vi "GT Get Sts Ext Mdl.vi"(7 "pStatus":u16, 8 "error in (no error)":errorcluster caption="错误输入（无错误）", 9 "chn":i16, 10 "mdl":i16, 11 "cardNum":i16) -> (0 "error out":errorcluster caption="错误输出", 3 "function return":i16, 5 "pStatus out":u16)   [LabVIEW 2014, in "gts.lvlib"]
doc: "GT_API GT_GetStsExtMdl(short cardNum,short mdl,short chn,unsigned short *pStatus);"
uses:
  gts.lvlib
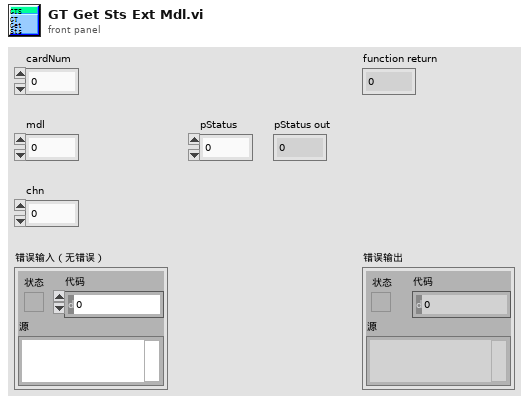
[diagram p1: front panel]
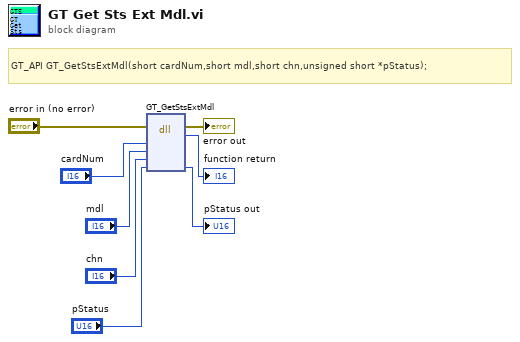
[diagram p0: block diagram]
diagram:
  # "GT_API GT_GetStsExtMdl(short cardNum,short mdl,short chn,unsigned short *pStatus);"
  n1 = dll-call lib="PTH2habs D固高科技资料GTS控制卡GTS卡18年上半年资料dllVC32bit\nmulti_cardgts.*" fn="GT_GetStsExtMdl"(error in="error in (no error)", "cardNum"="cardNum", "mdl"="mdl", "chn"="chn", "pStatus"="pStatus") -> (error out=→"error out":errorcluster, →"function return":i16, "pStatus"=→"pStatus out":u16)  [unwired: 5 in, 1 out]
